vi "Get Refnum by URL.vi"(8 "error in (no error)":errorcluster, 10 "URL":refnum<k21>, 11 "Map In":variant) -> (0 "error out":errorcluster, 1 "Found?":bool, 2 "Control Refnum":refnum<vi>, 3 "Map Out":variant)   [LabVIEW 2024]
doc: "Gets the control refnum from the map."
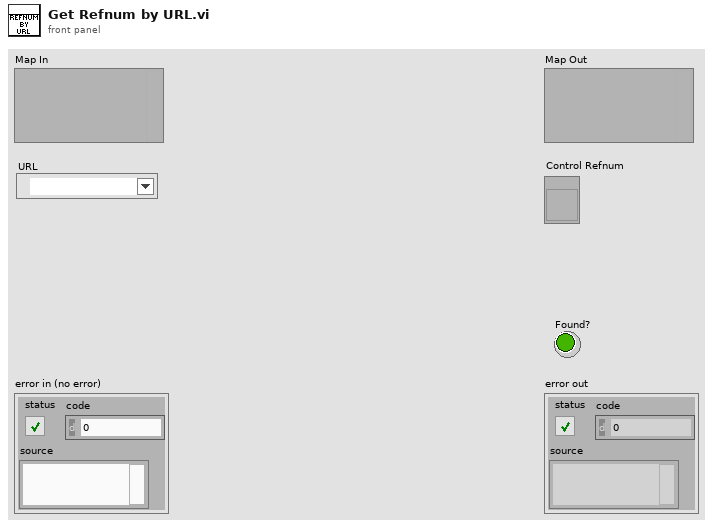
[diagram p1: front panel]
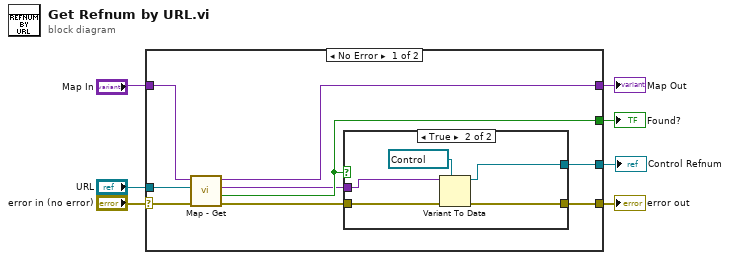
[diagram p0: block diagram]
diagram:
  n1 = case shown="No Error" "error in (no error)" {
    selector: "error in (no error)" -> [w14 w24]
    tunnel: [w15 w24] -> w6
    tunnel: [w13 w23] -> w5
    tunnel: "Map In" -> [w12 w23]
    tunnel: "URL" -> [w11 _]
    tunnel: [w10 _] -> w2
    tunnel: [w8 _] -> w1
    frame No Error {
      n2 = call "Map - Get.vi"("error in (no error)"=w14, "Key"=w11, "Map In"=w12) -> ("error out"=w16:errorcluster, "Found?"=w10:bool, "Value"=w9:variant, "Map Out"=w13:variant)  [unwired: 5 in]
      n3 = case shown="True" w10 {
        tunnel: w16 -> [w17 w21]
        tunnel: [w17 w20] -> w15
        tunnel: w9 -> [_ w19]
        tunnel: [_ w18] -> w8
        frame False {
        }
        frame True {
          n4 = Variant To Data(error in=w21, type=refnum<vi> refnum ("Ctl Refnum"), Variant=w19) -> (data=w18:refnum<vi>, error out=w20:errorcluster)
        }
      }
    }
    frame Error {
    }
  }
  "error out" <- w6
  "Map Out" <- w5
  "Found?" <- w2
  "Control Refnum" <- w1
